vi "Read Core Actors.vi"(11 "Base Attributes in":refnum<class "Base Attributes.lvclass">) -> (2 "Core Actors":refnum<class "Actor.lvclass">[](array[class]))   [LabVIEW 2025, in "jettl.lvlib" / "Base Attributes.lvlib" / "Base Attributes.lvclass"]
uses:
  Base Attributes.lvclass
  Actor/Actor.lvclass
  Base Attributes.lvclass/Base Attributes.ctl
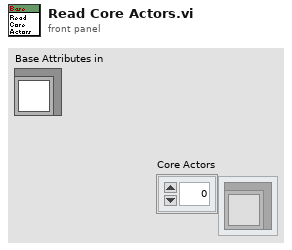
[diagram p1: front panel]
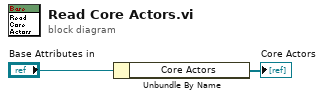
[diagram p0: block diagram]
diagram:
  n1 = Unbundle By Name("Base Attributes in") -> ("Core Actors"=→"Core Actors":refnum<class "Actor.lvclass">[])
